vi "Get All Connected Clients.vi"(8 "error in (no error)":errorcluster, 11 "Function in":refnum<class "Function.lvclass">) -> (0 "error out":errorcluster, 2 "Array of Connected Clients":T1[](array[typedef]), 3 "Function out":refnum<class "Function.lvclass">)   [LabVIEW 2016, in "Function Actor.lvlib" / "Function.lvclass"]
uses:
  <userlib>/Common Components/Function Actor/Function.lvclass
  <userlib>/Common Components/Common/Connection Cluster.ctl
  <userlib>/Common Components/Common/Connected Client Cluster.ctl
  <userlib>/Common Components/Function Actor/Function.lvclass/Function.ctl
  <userlib>/Common Components/Common/Common.lvlib
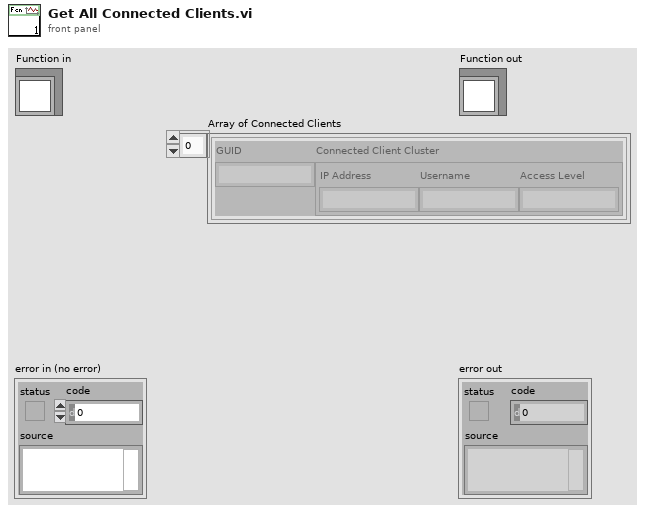
[diagram p1: front panel]
types:
  T1 = typedef "Common.lvlib/Connection Cluster.ctl" = cluster{"GUID":string, "Connected Client Cluster":T2}
  T2 = typedef "Common.lvlib/Connected Client Cluster.ctl" = cluster{"IP Address":string, "Username":string, "Access Level":string}
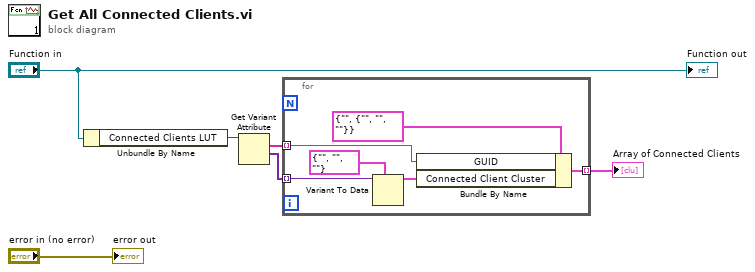
[diagram p0: block diagram]
diagram:
  n1 = Unbundle By Name("Function in") -> ("Connected Clients LUT"=w4:variant)
  n2 = Get Variant Attribute(Variant=w4) -> (names=w3:string[], values=w2:variant[])  [unwired: 3 in, 2 out]
  n3 = for {
    tunnel: w3 -> [w9] mode=indexing
    tunnel: w2 -> [w12] mode=indexing
    tunnel: [w7] -> w1 mode=indexing
    n4 = Variant To Data(type=T2 {"IP Address"="", "Username"="", "Access Level"=""} ("Connected Client Cluster"), Variant=w12) -> (data=w8:T2)  [unwired: 1 in, 1 out]
    n5 = Bundle By Name(cluster=T1 {"GUID"="", "Connected Client Cluster"={"IP Address"="", "Username"="", "Access Level"=""}} ("Connection Cluster"), "GUID"=w9, "Connected Client Cluster"=w8) -> (w7:T1)
  }
  "Array of Connected Clients" <- w1
  "error out" <- "error in (no error)"
  "Function out" <- "Function in"
